vi "Configure TTL.vi"(0 "VISA resource name":refnum<visa-resource-name>, 1 "TTL4 Polarity (0: Active High)":i32(ring) items=["Active High", "Active Low"], 2 "TTL2 Level (F: Disable)":bool, 3 "TTL4 Level (F: Disable)":bool, 5 "TTL1 Polarity (0: Active High)":i32(ring) items=["Active High", "Active Low"], 7 "TTL2 Polarity (0: Active High)":i32(ring) items=["Active High", "Active Low"], 9 "TTL3 Polarity (0: Active High)":i32(ring) items=["Active High", "Active Low"], 11 "error in (no error)":errorcluster, 12 "TTL1 Level (F: Disable)":bool, 13 "TTL3 Level (F: Disable)":bool) -> (4 "VISA resource name out":refnum<visa-resource-name>, 15 "error out":errorcluster)   [LabVIEW 2016, in "Keithley 6517.lvlib"]
doc: "Sets the polarity and controls the digital output of lines 1 through 4.\n\n<B>Note:</B>\nThis VI is <B>NOT</B> compatible with model <B>6514</B>."
uses:
  <instrlib>/Keithley 6517/Keithley 6517.lvlib
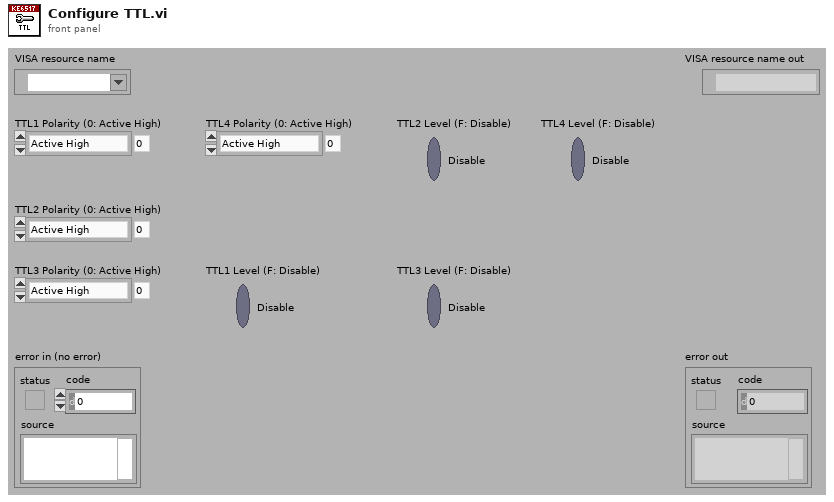
[diagram p1: front panel]
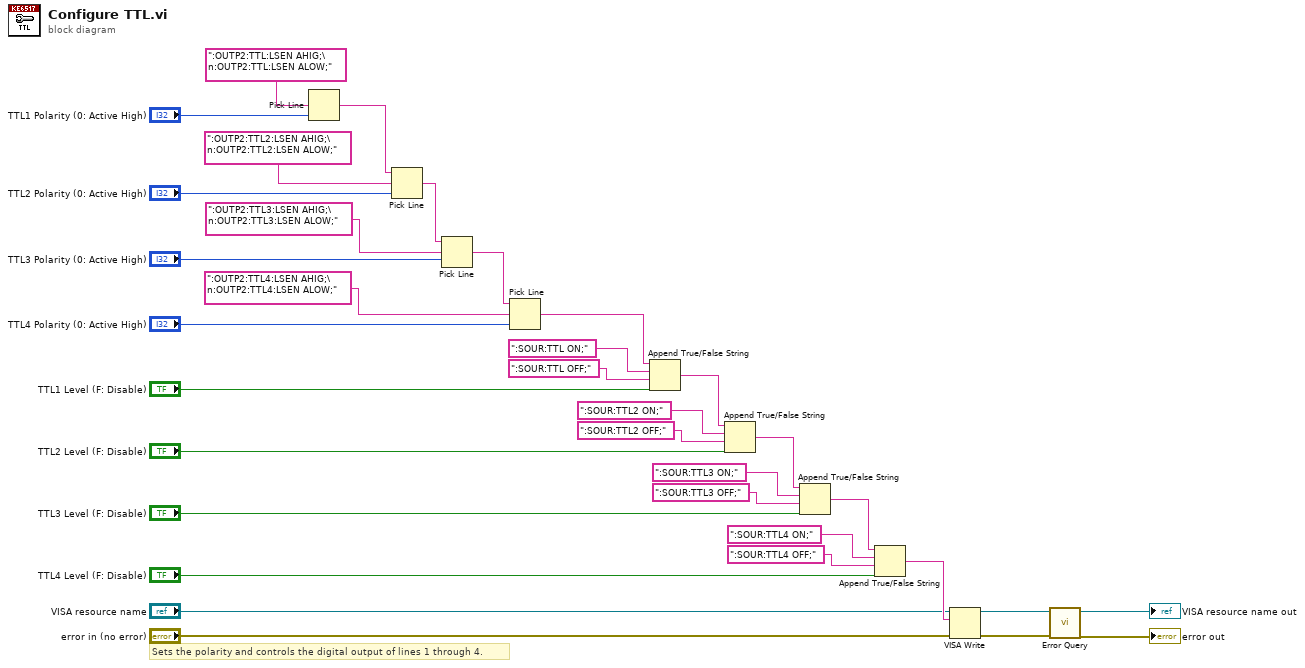
[diagram p0: block diagram]
diagram:
  # "Sets the polarity and controls the digital output of lines 1 through 4."
  n1 = Pick Line(multi-line string=":OUTP2:TTL:LSEN AHIG;\n:OUTP2:TTL:LSEN ALOW;", line index="TTL1 Polarity (0: Active High)") -> (output string=w9:string)  [unwired: 1 in]
  n2 = Pick Line(string ("")=w9, multi-line string=":OUTP2:TTL2:LSEN AHIG;\n:OUTP2:TTL2:LSEN ALOW;", line index="TTL2 Polarity (0: Active High)") -> (output string=w5:string)
  n3 = Pick Line(string ("")=w5, multi-line string=":OUTP2:TTL3:LSEN AHIG;\n:OUTP2:TTL3:LSEN ALOW;", line index="TTL3 Polarity (0: Active High)") -> (output string=w3:string)
  n4 = Pick Line(string ("")=w3, multi-line string=":OUTP2:TTL4:LSEN AHIG;\n:OUTP2:TTL4:LSEN ALOW;", line index="TTL4 Polarity (0: Active High)") -> (output string=w1:string)
  n5 = Append True/False String(1:"TTL1 Level (F: Disable)", 2:":SOUR:TTL OFF;", 3:":SOUR:TTL ON;", 4:w1) -> (0:w31:string)
  n6 = Append True/False String(1:"TTL2 Level (F: Disable)", 2:":SOUR:TTL2 OFF;", 3:":SOUR:TTL2 ON;", 4:w31) -> (0:w27:string)
  n7 = Append True/False String(1:"TTL3 Level (F: Disable)", 2:":SOUR:TTL3 OFF;", 3:":SOUR:TTL3 ON;", 4:w27) -> (0:w23:string)
  n8 = Append True/False String(1:"TTL4 Level (F: Disable)", 2:":SOUR:TTL4 OFF;", 3:":SOUR:TTL4 ON;", 4:w23) -> (0:w19:string)
  n9 = VISA Write(VISA resource name="VISA resource name", write buffer=w19, error in (no error)="error in (no error)") -> (VISA resource name out=w16:refnum<visa-resource-name>, error out=w15:errorcluster)  [unwired: 1 out]
  n10 = call <instrlib>:"Error Query.vi"("error in (no error)"=w15, "VISA resource name"=w16) -> ("error out"=→"error out":errorcluster, "VISA resource name out"=→"VISA resource name out":refnum<visa-resource-name>)  [unwired: 6 in, 2 out]
